vi "Set LED (Boolean).vi"(8 "error in (no error)":errorcluster, 9 "Enable":bool, 10 "LED Selector":T1, 11 "LINX-AutomationHat in":refnum<class "LINX-AutomationHat.lvclass">) -> (0 "error out":errorcluster, 3 "LINX-AutomationHat out":refnum<class "LINX-AutomationHat.lvclass">)   [LabVIEW 2020, in "LINX-AutomationHat.lvclass"]
doc: "Sets the LED on/off according to the default brightness setting."
uses:
  LINX-AutomationHat.lvclass
  LEDs.ctl
  LINX-SN3218/LINX-SN3218.lvclass
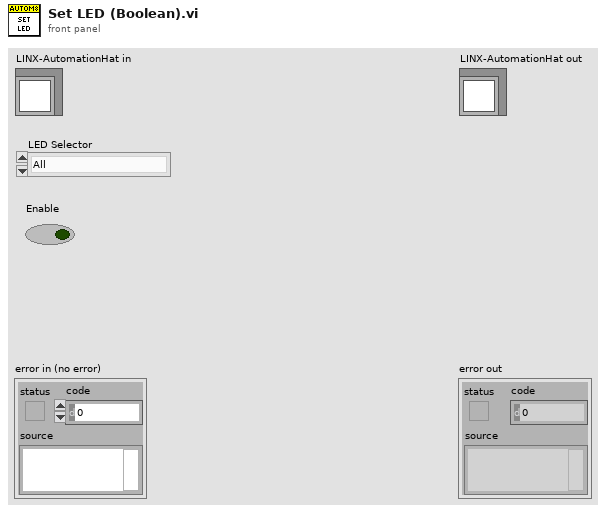
[diagram p1: front panel]
types:
  T1 = typedef "LINX-AutomationHat.lvclass/LEDs.ctl" = enum16{"All", "ADC1", "ADC2", "ADC3", "Output1", "Output2", "Output3", "Relay1NO", "Relay1NC", "Relay2NO", "Relay2NC", "Relay3NO", "Relay3NC", "Input3", "Input2", "Input1", "Warn", "Comms", "Power"}
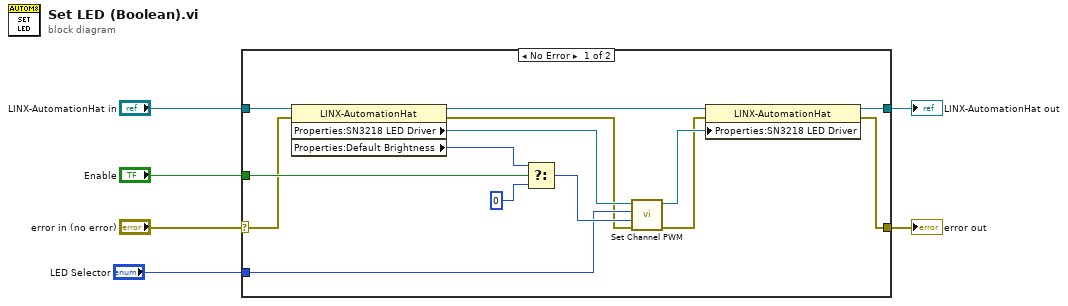
[diagram p0: block diagram]
diagram:
  n1 = case shown="No Error" "error in (no error)" {
    selector: "error in (no error)" -> [w8 w22]
    tunnel: [w9 w22] -> w5
    tunnel: [w12 w21] -> w3
    tunnel: "LINX-AutomationHat in" -> [w20 w21]
    tunnel: "Enable" -> [w16 _]
    tunnel: "LED Selector" -> [w14 _]
    frame No Error {
      n2 = property class="LINX-AutomationHat"(reference=w20, error in=w8) -> (reference out=w13:refnum<class "LINX-AutomationHat.lvclass">, error out=w7:errorcluster, "Properties:SN3218 LED Driver"=w19:refnum<class "LINX-SN3218.lvclass">, "Properties:Default Brightness"=w18:u8)
      n3 = Select(t=w18, s=w16, f=u8 0) -> (s? t:f=w17:u8)
      n4 = call "Set Channel PWM.vi"("error in (no error)"=w7, "PWM (0-255)"=w17, "LED Channel (0-18, 0=all)"=w14, "LINX-SN3218 in"=w19) -> ("error out"=w10:errorcluster, "LINX-SN3218 out"=w11:refnum<class "LINX-SN3218.lvclass">)  [unwired: 6 in]
      n5 = property class="LINX-AutomationHat"(reference=w13, error in=w10, "Properties:SN3218 LED Driver"=w11) -> (reference out=w12:refnum<class "LINX-AutomationHat.lvclass">, error out=w9:errorcluster)
    }
    frame Error {
    }
  }
  "error out" <- w5
  "LINX-AutomationHat out" <- w3
